vi "GetUnorderedList.vi"(8 "error in (no error)":errorcluster, 11 "OrderedList in":refnum<class "UnorderedList.lvclass">) -> (0 "error out":errorcluster, 2 "OrderedList":refnum<class "Collection.lvclass">, 3 "OrderedList out":refnum<class "UnorderedList.lvclass">)   [LabVIEW 2021, in "Markdown.lvlib" / "UnorderedList.lvclass"]
uses:
  UnorderedList.lvclass
  Collection/Collection.lvclass
  UnorderedList.lvclass/UnorderedList.ctl
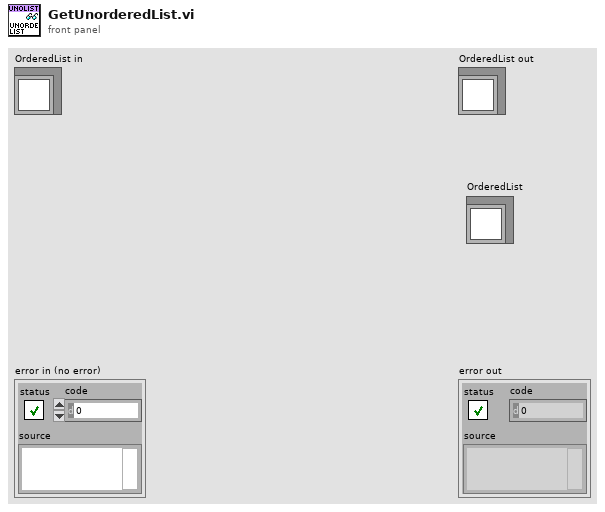
[diagram p1: front panel]
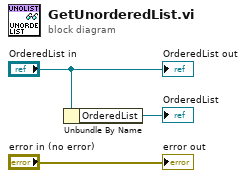
[diagram p0: block diagram]
diagram:
  n1 = Unbundle By Name("OrderedList in") -> ("OrderedList"=→"OrderedList":refnum<class "Collection.lvclass">)
  "error out" <- "error in (no error)"
  "OrderedList out" <- "OrderedList in"
